vi "test-tdms read.vi"() -> ()   [LabVIEW 2014]
uses:
  <vilib>/rvi/interface/nirviOpenFPGA/nirviOpenFPGA.xnode
  FPGA Bitfiles/mySynth_FPGATarget_FPGAMain_WASpsvx+XwM.lvbitx
  FPGA Main.vi
  <vilib>/FPGAPlugInAG/myRIO-1900/niLvFpga_Open_myRIO-1900.vi
  <vilib>/rvi/interface/common/dynamic/niFpgaDynamicAddResources.vi
  <vilib>/rvi/interface/nirviCloseFPGA/nirviCloseFPGA.xnode
  <vilib>/FPGAPlugInAG/Dynamic/niLvFpga_Close_Dynamic.vi
  Controls/Track Enable.ctl
panel:
  in  "error in":errorcluster
  out "error out":errorcluster
  in  "stop":bool
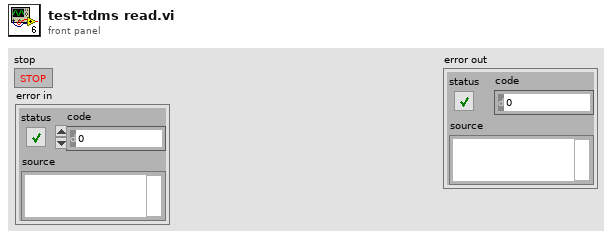
[diagram p1: front panel]
types:
  T1 = typedef "Track (File) References.ctl" = cluster{"Track_1_Ref":refnum<k34>, "Track_2_Ref":refnum<k34>, "Track_3_Ref":refnum<k34>, "Track_4_Ref":refnum<k34>, "Track_Name_1":string, "Track_Name_2":string, "Track_Name_3":string, "Track_Name_4":string}
  T2 = typedef "Track Enable.ctl" = cluster{"Track_1 _Enable ":bool, "Track_2 _Enable ":bool, "Track_3 _Enable ":bool, "Track_4 _Enable ":bool}
  T3 = typedef "4 Track Audio.ctl" = cluster{"Track 0":T4, "Track 1":T4, "Track 2":T4, "Track 3":T4}
  T4 = typedef "Audio In.ctl" = cluster{"AudioIn/Left (N Samples)":i16[], "AudioIn/Right (N Samples)":i16[]}
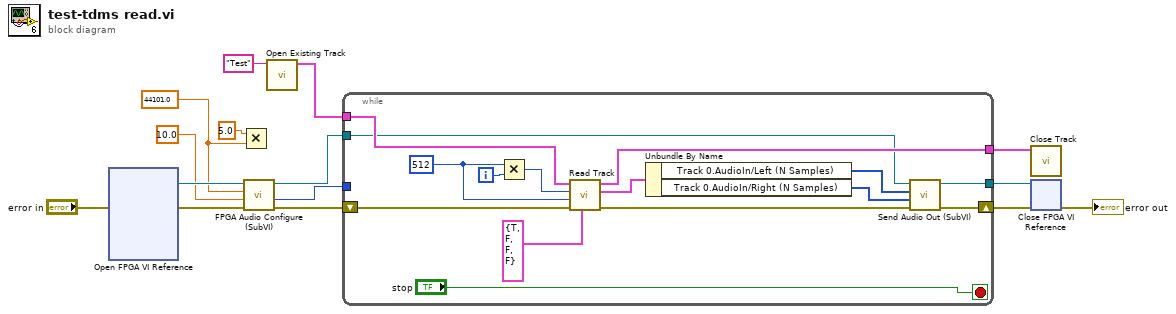
[diagram p0: block diagram]
diagram:
  w7 = 44101.0 ("Audio Sample Rate (Hz)")
  n1 = xnode "Open FPGA VI Reference"("error in"="error in") -> ("FPGA VI Reference Out"=w15:refnum<k20>, "error out"=w9:errorcluster)  [unwired: 1 in]
  n2 = Multiply(x=5.0, y=w7) -> ()  [unwired: 1 out]
  n3 = call "FPGA Audio Configure (SubVI).vi"("error in (no error)"=w9, "Read Rate (Hz)"=10.0, "Audio Sample Rate (Hz)"=w7, "Refnum in"=w15) -> ("error out"=w11:errorcluster, "Required loop period (ms)"=w8:u32, "Refnum out"=w5:refnum<k20>)  [unwired: 4 in, 1 out]
  n4 = call "Open Existing Track.vi"("Track Name"="Test") -> ("Track (File) References"=w3:T1)  [unwired: 9 in, 1 out]
  n5 = while {
    shift-right: [w20] -> w13
    shift-left: w11 -> [w25]
    tunnel: w8 -> [_]
    tunnel: w5 -> [w22]
    tunnel: w3 -> [w28]
    tunnel: [w23] -> w2
    tunnel: [w21] -> w1
    i -> [w29]
    stop <- "stop" stop-if-true
    w26 = 512
    n6 = Multiply(x=w26, y=w29) -> (x*y=w27:i32)
    n7 = call "Read Track.vi"(6:T2 {"Track_1 _Enable "=TRUE, "Track_2 _Enable "=FALSE, "Track_3 _Enable "=FALSE, "Track_4 _Enable "=FALSE} ("Track Enable"), "Error In"=w25, "Number Of Elements to Read"=w26, "Read Position"=w27, "Track (File) References In"=w28) -> ("Error Out"=w19:errorcluster, "4-Track Audio"=w18:T3, "Track (File) References Out"=w23:T1)  [unwired: 4 in]
    n8 = Unbundle By Name(w18) -> ("Track 0.AudioIn/Left (N Samples)"=w17:i16[], "Track 0.AudioIn/Right (N Samples)"=w16:i16[])
    n9 = call "Send Audio Out (SubVI).vi"("error in (no error)"=w19, "Right Audio Out"=w16, "Left Audio Out"=w17, "Refnum in"=w22) -> ("error out"=w20:errorcluster, "Refnum out"=w21:refnum<k20>)  [unwired: 6 in]
  }
  n10 = call "Close Track.vi"("Track (File) References"=w2) -> ()  [unwired: 10 in, 1 out]
  n11 = xnode "Close FPGA VI Reference"("FPGA VI Reference In"=w1, "error in"=w13) -> ("error out"=→"error out":errorcluster)
